vi "PNA_CalFile_Check.vi"(0 "PNA_IN":refnum<visa-resource-name>="TCPIP0::169.254.70.180::inst0::INSTR", 1 "RF_SW_IN":refnum<visa-resource-name>="GPIB0::29::INSTR", 3 "PNA_file Path":string="D:\\State Files\\WAM_PRODUCTION.csa", 5 "error in":errorcluster, 7 "HrsToFlag":dbl=24.0, 8 "PopUp Alert(t)":bool, 9 "RunFileCheck(t)":bool=TRUE, 11 "RunCalCheck(t)":bool=TRUE, 13 "DoCal(t)":bool=TRUE) -> (6 "File Date/Time":string="12:07:34 03/13/2023 ", 10 "Cal_Flag(t)":bool=TRUE, 19 "error out":errorcluster)   [LabVIEW 2018]
uses:
  Instruments/PNA-X/PNA-X.lvlib
  Instruments/PNA/lib functions/Agilent ENA Series.lvlib
panel:
  out "Success?(t)":bool=TRUE
  out "CalMessage":string="The Calibration / State File \" D:\\State Files\\WAM_PRODUCTION.csa\" is more than 0.01 Hours old. \rA Re-Calibration is required"
  in  "Clear PNA Errors(t)":bool=TRUE
  out "file exists?(t)":bool=TRUE
  out "PNA_VISA(T)":bool=TRUE
  out "RF_SW_VISA(T)":bool=TRUE
  out "system time(str)":string="14:25:52 03/13/2023"
  # "PRESS NEXT TO DO A CALIBRATION \n...TAKES ABOUT 3 Seconds"
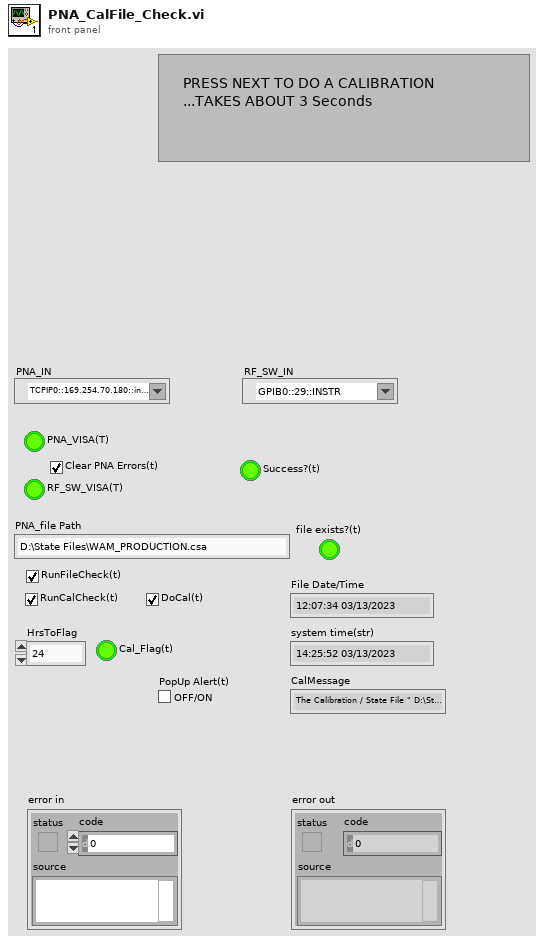
[diagram p1: front panel]
types:
  T1 = enum32{"Invalid", "Standard", "Closed", "Hidden", "Minimized", "Maximized"}
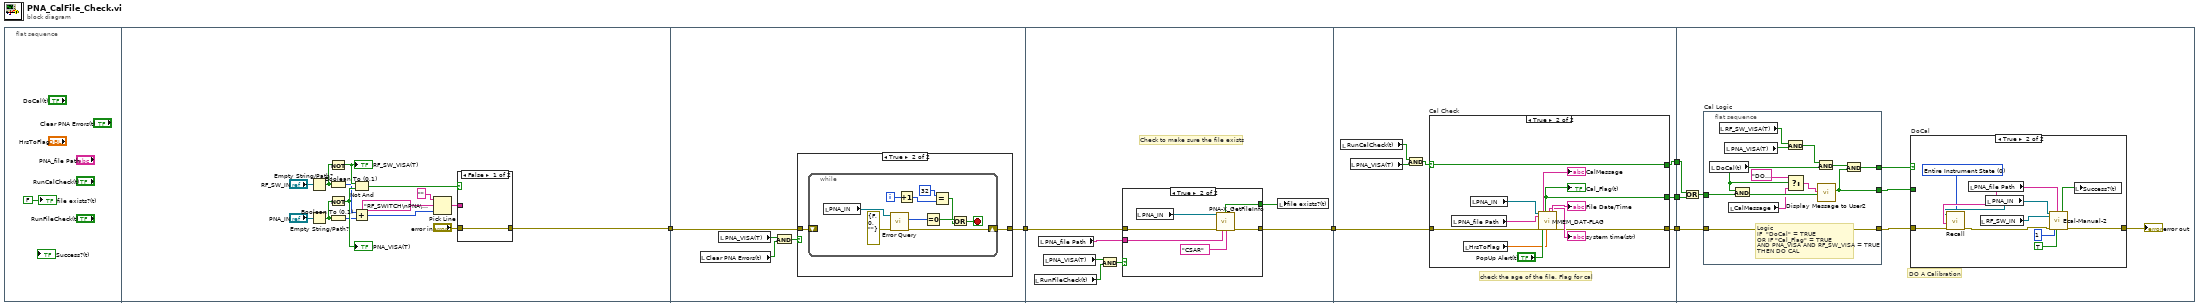
[diagram p0: block diagram]
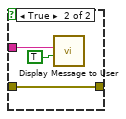
[diagram p2: hidden frame]
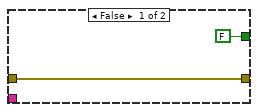
[diagram p4: hidden frame]
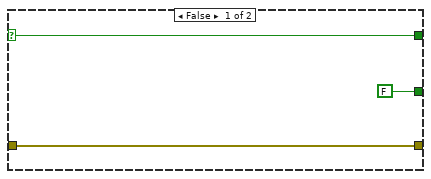
[diagram p5: hidden frame]
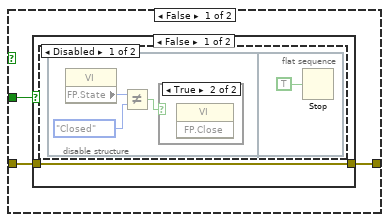
[diagram p6: hidden frame]
diagram:
  n1 = flat-sequence {
    tunnel: [w18] -> w3
    tunnel: w3 -> [w30]
    tunnel: [w31] -> w2
    tunnel: [w50] -> w6
    tunnel: w2 -> [w51]
    tunnel: w6 -> [w66]
    tunnel: [w65] -> w5
    tunnel: [w64] -> w4
    tunnel: [w60] -> w1
    tunnel: w5 -> [w87]
    tunnel: w4 -> [w83]
    tunnel: w1 -> [w84]
    frame #0 {
      "file exists?(t)" <- FALSE
    }
    frame #1 {
      n2 = Empty String/Path?(string/path="RF_SW_IN") -> (empty?=w15:bool)
      n3 = Empty String/Path?(string/path="PNA_IN") -> (empty?=w14:bool)
      n4 = Not(x=w15) -> (.not. x?=w22:bool)
      "RF_SW_VISA(T)" <- w22
      n5 = Boolean To (0,1)(Boolean=w15) -> (0, 1=w12:i16)
      n6 = Not(x=w14) -> (.not. x?=w21:bool)
      "PNA_VISA(T)" <- w21
      n7 = Boolean To (0,1)(Boolean=w14) -> (0, 1=w13:i16)
      n8 = Add(x=w12, y=w13) -> (x+y=w10:i16)
      n9 = Not And(1:w21, 2:w22) -> (0:w20:bool)
      n10 = Pick Line(string ("")="", multi-line string="RF_SWITCH\nPNA\nRF_SWITCH AND PNA ", line index=w10) -> (output string=w8:string)
      n11 = case shown="False" w20 {
        tunnel: "error in" -> [w23 w25]
        tunnel: [w23 w25] -> w18
        tunnel: w8 -> [_ w26]
        frame False {
        }
        frame True {
          n12 = call "Display Message to User"("Enable"=TRUE, "Message"=w26) -> ()  [unwired: 8 in, 2 out]
        }
      }
    }
    frame #2 {
      n13 = local read "Clear PNA Errors(t)"() -> (w29:bool)
      n14 = local read "PNA_VISA(T)"() -> (w27:bool)
      n15 = And(x=w27, y=w29) -> (x .and. y?=w28:bool)
      n16 = case shown="True" w28 {
        tunnel: [w32 w34] -> w31
        tunnel: w30 -> [w32 w33]
        frame False {
        }
        frame True {
          n17 = while {
            shift-right: [w36] -> w34
            shift-left: w33 -> [_]
            i -> [w40]
            stop <- w41 stop-if-true
            n18 = local read "PNA_IN"() -> (w44:refnum<visa-resource-name>)
            n19 = call "Error Query.vi"("error in (no error)"=errorcluster {"status"=FALSE, "code"=0, "source"=""}, "VISA Resource Name"=w44) -> ("error out"=w36:errorcluster, "Error"=w42:i32)  [unwired: 4 in, 2 out]
            n20 = Increment(x=w40) -> (x+1=w37:i32)
            n21 = Equal To 0?(x=w42) -> (x = 0?=w43:bool)
            n22 = Equal?(x=32, y=w37) -> (x = y?=w39:bool)
            n23 = Or(x=w43, y=w39) -> (x .or. y?=w41:bool)
          }
        }
      }
    }
    frame #3 {
      # "Check to make sure the file exists"
      n24 = local read "RunFileCheck(t)"() -> (w49:bool)
      n25 = local read "PNA_file Path"() -> (w45:string)
      n26 = local read "PNA_VISA(T)"() -> (w46:bool)
      n27 = And(x=w46, y=w49) -> (x .and. y?=w47:bool)
      n28 = case shown="True" w47 {
        tunnel: w51 -> [w53 w59]
        tunnel: [w53 w57] -> w50
        tunnel: w45 -> [_ w56]
        tunnel: [FALSE ("file exists?(t)") w54] -> w48
        frame False {
        }
        frame True {
          n29 = local read "PNA_IN"() -> (w55:refnum<visa-resource-name>)
          n30 = call "PNA-X_GetFileInfo.vi"("VISA IN"=w55, "error in"=w59, "Path"=w56, "Types"="CSAR") -> ("file exists?(t)"=w54:bool, "error out"=w57:errorcluster)  [unwired: 8 in, 2 out]
        }
      }
      n31 = local write "file exists?(t)"(w48) -> ()
    }
    frame #4 {
      # "check the age of the file, Flag for cal"
      n32 = local read "RunCalCheck(t)"() -> (w63:bool)
      n33 = local read "PNA_VISA(T)"() -> (w61:bool)
      n34 = And(x=w63, y=w61) -> (x .and. y?=w62:bool)
      n35 = case "Cal Check" shown="True" w62 {
        selector: w62 -> [w67 w71]
        tunnel: w66 -> [w69 w80]
        tunnel: [FALSE ("=>SelectedHrs?(t)") w70] -> w65
        tunnel: [w69 w75] -> w64
        tunnel: [w67 w71] -> w60
        frame False {
        }
        frame True {
          n36 = local read "PNA_file Path"() -> (w74:string)
          n37 = local read "HrsToFlag"() -> (w73:dbl)
          n38 = local read "PNA_IN"() -> (w76:refnum<visa-resource-name>)
          n39 = call "MMEM_DAT-FLAG.vi"("PNA IN"=w76, "FilePath"=w74, "error in"=w80, "PopUp Alert(t)"="PopUp Alert(t)", "HrsToFlag"=w73) -> ("CalMessage"=→"CalMessage":string, "=>SelectedHrs?(t)"=w70:bool, "system time(str)"=→"system time(str)":string, "File Time/Date Out (Str)"=→"File Date/Time":string, "error out"=w75:errorcluster)  [unwired: 9 in, 1 out]
          "Cal_Flag(t)" <- w70
        }
      }
    }
    frame #5 {
      # "DO A Calibration"
      n40 = Or(x=w84, y=w87) -> (x .or. y?=w85:bool)
      n41 = flat-sequence "Cal Logic" {
        tunnel: w85 -> [w97]
        tunnel: [w96] -> w86
        tunnel: w83 -> [w95]
        tunnel: [w95] -> w82
        tunnel: [w94] -> w81
        frame #0 {
          # "Logic\nIF  \"DoCal\" = TRUE\nOR IF \"Cal_Flag\" = TRUE\nAND PNA_VISA AND RF_SW_VISA = TRUE\nTHEN DO CAL"
          n42 = local read "DoCal(t)"() -> (w92:bool)
          n43 = local read "RF_SW_VISA(T)"() -> (w100:bool)
          n44 = local read "PNA_VISA(T)"() -> (w101:bool)
          n45 = local read "CalMessage"() -> (w91:string)
          n46 = And(x=w92, y=w97) -> (x .and. y?=w93:bool)
          n47 = And(x=w100, y=w101) -> (x .and. y?=w99:bool)
          n48 = Select(t="DO Calibration = TRUE; A Calibration is required", s=w92, f=w91) -> (s? t:f=w90:string)
          n49 = And(x=w99, y=w92) -> (x .and. y?=w98:bool)
          n50 = call "Display Message to User2"("Enable"=w93, "Message"=w90) -> ("OK"=w94:bool)  [unwired: 8 in, 1 out]
          n51 = And(x=w98, y=w94) -> (x .and. y?=w96:bool)
        }
      }
      n52 = case "DoCal" shown="True" w86 {
        tunnel: w82 -> [w104 w114]
        tunnel: [w103 w119] -> w88
        tunnel: w81 -> [w102 _]
        frame False {
          n53 = case shown="False" w102 {
            tunnel: w104 -> [w105 w110]
            tunnel: [w105 w110] -> w103
            frame False {
              n54 = disable-structure shown="Disabled" {
                frame Disabled {
                  n55 = flat-sequence {
                    frame #0 {
                      n56 = property class="VI"() -> ("FP.State"=w108:T1)  [unwired: 2 in, 2 out]
                      n57 = Not Equal?(x=w108, y=T1."Closed") -> (x != y?=w106:bool)
                      n58 = case shown="True" w106 {
                        frame False {
                        }
                        frame True {
                          n59 = invoke class="VI" method="FP.Close"() -> ()  [unwired: 3 in, 3 out]
                        }
                      }
                    }
                    frame #1 {
                      n60 = Stop(stop? (T)=TRUE) -> ()
                    }
                  }
                }
                frame Enabled {
                }
              }
            }
            frame True {
            }
          }
        }
        frame True {
          w111 = u16 0 items=["Entire Instrument State", "Segment Sweep Table", "Limit Table", "Power Sensor A", "Power Sensor B", "VBA Project", "Loss Compensation Table 1", "Loss Compensation Table 2", "Loss Compensation Table 3", "Loss Compensation Table 4", "Ripple Limit Table"] ("Data Type (0: Entire Instrument State)")
          n61 = local read "PNA_file Path"() -> (w113:string)
          n62 = local read "RF_SW_IN"() -> (w120:refnum<visa-resource-name>)
          n63 = local read "PNA_IN"() -> (w112:refnum<visa-resource-name>)
          n64 = call "Recall.vi"("error in (no error)"=w114, "File Name ()"=w113, "Data Type (0: Entire Instrument State)"=w111, "VISA resource name"=w112) -> ("error out"=w115:errorcluster)  [unwired: 6 in, 1 out]
          n65 = call "Ecal-Manual-2.vi"("PNA_IN"=w112, "RF_Switch_In"=w120, "error in"=w115, "Channel"=1, "RecallFile"=w113, "Save to File(t)"=TRUE) -> ("Success?(t)"=w116:bool, "error out"=w119:errorcluster)  [unwired: 10 in, 2 out]
          n66 = local write "Success?(t)"(w116) -> ()
        }
      }
      "error out" <- w88
    }
  }
